vi "apply.all.available.storeDates.vi"() -> ()   [LabVIEW 2024]
uses:
  CV_Shared_Library/CV_Shared_Library.lvlib
  <vilib>/addons/_JKI.lib/Serialization/JSON/JKI JSON Serialization.lvlib
panel:
  out "current volume":string
  out "error out":errorcluster
  out "progress":i32(slide) scale=0.0..4694.0
  in  "Volumes Path":path
  in  "Issues Path":path
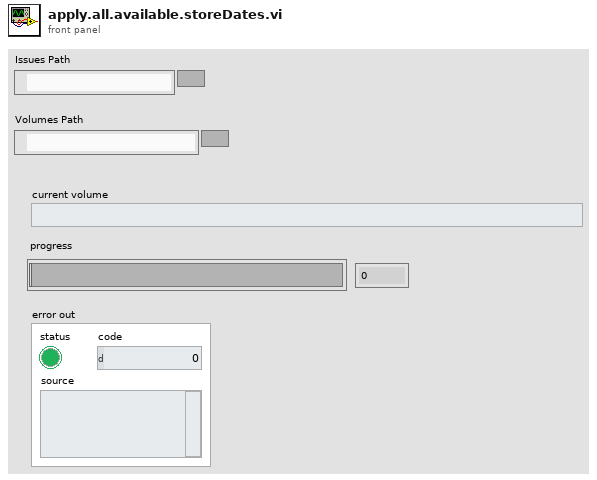
[diagram p1: front panel]
types:
  T1 = typedef "local_issue.ctl" = cluster{"cover_date":timestamp, "id":i32, "cv_id":string, "name":string, "sortable_name":string, "issue_number":string, "deck":string, "description":string, "volume":T2, "store_date":timestamp, "date_last_updated":timestamp, "site_detail_url":string, "cover_url":string, "associated_images":T3[], "characters":T2[], "concepts":T2[], "creators":T4[], "storyArcs":T2[], "teams":T2[]}
  T2 = typedef "comicvine_issue.generic_credit.ctl" = cluster{"id":i32, "name":string}
  T3 = typedef "comicvine_issue.associated_image.ctl" = cluster{"original_url":string, "id":i32}
  T4 = typedef "comicvine_issue.person_credit.ctl" = cluster{"id":i32, "name":string, "role":string}
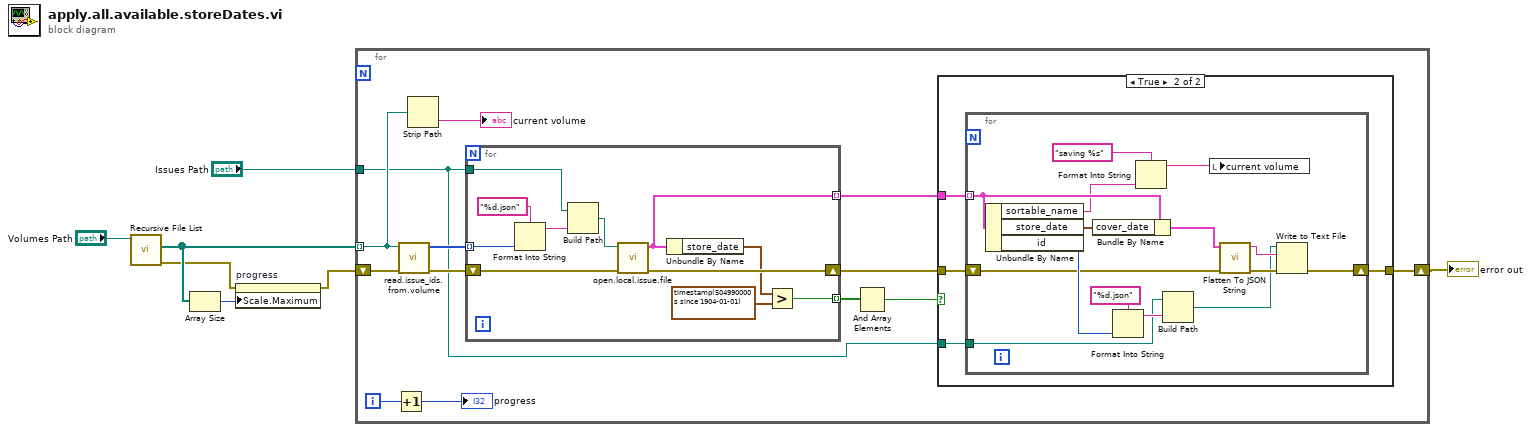
[diagram p0: block diagram]
diagram:
  n1 = call <vilib>:"Recursive File List.vi"("Folder Path"="Volumes Path") -> ("error out"=w4:errorcluster, "All Files in Dir"=w5:path[])  [unwired: 6 in, 3 out]
  n2 = Array Size(array=w5) -> (size(s)=w6:i32)
  n3 = property on="progress" class="Slide (strict)"(error in=w4, "Scale.Maximum"=w6) -> (error out=w3:errorcluster)  [unwired: 1 in, 1 out]
  n4 = for {
    tunnel: w5 -> [w15] mode=indexing
    shift-right: [w10] -> w1
    shift-left: w3 -> [w18]
    tunnel: "Issues Path" -> [w8]
    i -> [w20]
    n5 = Increment(x=w20) -> (x+1=→"progress":i32)
    n6 = call "read.issue_ids.from.volume.vi"("error in"=w18, "file (use dialog)"=w15) -> ("error out"=w16:errorcluster, "issue_ids"=w17:i32[])  [unwired: 8 in]
    n7 = Strip Path(path=w15) -> (name=→"current volume":string)  [unwired: 1 out]
    n8 = for {
      tunnel: w17 -> [w50] mode=indexing
      shift-right: [w45] -> w11
      shift-left: w16 -> [w46]
      tunnel: w8 -> [w48]
      tunnel: [w42] -> w13 mode=indexing
      tunnel: [w41] -> w9 mode=indexing
      n9 = Format Into String(format string="%d.json", w50) -> (resulting string=w49:string)  [unwired: 2 in, 1 out]
      n10 = Build Path(base path=w48, name or relative path=w49) -> (appended path=w47:path)
      n11 = call "open.local.issue.file.vi"("error in (no error)"=w46, "volume json"=w47) -> ("error out"=w45:errorcluster, "issue"=w41:T1)  [unwired: 8 in]
      n12 = Unbundle By Name(w41) -> ("store_date"=w44:timestamp)
      n13 = Greater?(x=w44, y=timestamp(504990000 s since 1904-01-01)) -> (0:w42:bool)
    }
    n14 = And Array Elements(Boolean array=w13) -> (logical AND=w12:bool)
    n15 = case shown="True" w12 {
      tunnel: w11 -> [w21 w23]
      tunnel: [w21 w22] -> w10
      tunnel: w9 -> [_ w25]
      tunnel: w8 -> [_ w24]
      frame False {
      }
      frame True {
        n16 = for {
          tunnel: w25 -> [w40] mode=indexing
          tunnel: w24 -> [w35]
          shift-right: [w30] -> w22
          shift-left: w23 -> [w33]
          n17 = Unbundle By Name(w40) -> ("sortable_name"=w27:string, "store_date"=w39:timestamp, "id"=w37:i32)
          n18 = Bundle By Name(cluster=w40, "cover_date"=w39) -> (w34:T1)
          n19 = Format Into String(format string="%d.json", w37) -> (resulting string=w36:string)  [unwired: 2 in, 1 out]
          n20 = Format Into String(format string="saving %s", w27) -> (resulting string=w26:string)  [unwired: 2 in, 1 out]
          n21 = Build Path(base path=w35, name or relative path=w36) -> (appended path=w29:path)
          n22 = local write "current volume"(w26) -> ()
          n23 = call <vilib>:"Flatten To JSON String.vi"("error in"=w33, "Variant"=w34) -> ("error out"=w32:errorcluster, "JSON String"=w31:string)  [unwired: 8 in]
          n24 = Write to Text File(file (use dialog)=w29, text=w31, error in=w32) -> (error out=w30:errorcluster)  [unwired: 1 in, 2 out]
        }
      }
    }
  }
  "error out" <- w1
